vi "Set PCL Decimation.vi"(8 "error in (no error)":errorcluster, 10 "PCL decimation":u32=1, 11 "instrument addon refnum in":T1 format="%.0x") -> (0 "error out":errorcluster, 3 "instrument addon refnum":T1 format="%.0x")   [LabVIEW 2019, in "Instrument Addon Scripting API.lvlib"]
doc: "Assigns a new PCL decimation value to the specified Instrument Addon Custom Device."
uses:
  Instrument Addon Scripting API.lvlib
  <vilib>/NI VeriStand/Custom Device API/Custom Device Item Ref.ctl
  Addon/Addon Shared/SubVIs/Constants.vi
  <vilib>/NI/NI VeriStand Advanced SysDef API/_SubVIs/SysDef.Property.Set.U32.vi
  Addon/Addon Shared/Instrument Addon Shared.lvlib
  <vilib>/NI/NI VeriStand Advanced SysDef API/SysDef API/Advanced System Definition.lvlib
  <vilib>/NI VeriStand/Custom Device API/Custom Device API.lvlib
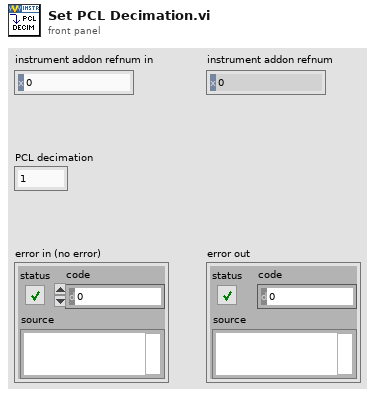
[diagram p1: front panel]
types:
  T1 = typedef "Custom Device API.lvlib/Custom Device Item Ref.ctl" = u64
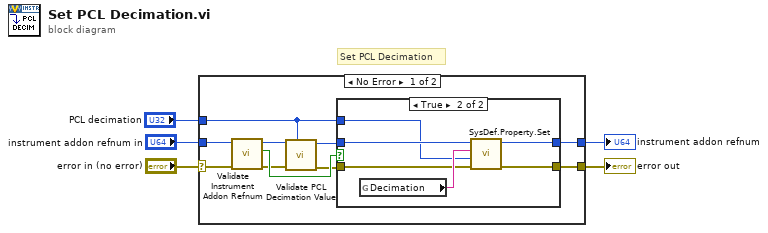
[diagram p0: block diagram]
diagram:
  # "Set PCL Decimation"
  n1 = case shown="No Error" "error in (no error)" {
    selector: "error in (no error)" -> [w11 w25]
    tunnel: "instrument addon refnum in" -> [w10 w24]
    tunnel: [w15 w25] -> w4
    tunnel: [w14 w24] -> w1
    tunnel: "PCL decimation" -> [w12 _]
    frame No Error {
      n2 = call "Validate Instrument Addon Refnum.vi"("Error In"=w11, "Refnum In"=w10) -> ("Error Out"=w8:errorcluster, "Is Instrument Addon?"=w13:bool, "Refnum Out"=w9:T1)  [unwired: 7 in]
      n3 = call "Validate PCL Decimation Value.vi"("PCL Decimation"=w12, "Error In"=w8, "Instrument Addon Refnum In"=w9) -> ("Error Out"=w7:errorcluster, "Instrument Addon Refnum Out"=w6:T1)  [unwired: 7 in]
      n4 = case shown="True" w13 {
        tunnel: w12 -> [_ w18]
        tunnel: [w16 w22] -> w15
        tunnel: [w17 w21] -> w14
        tunnel: w6 -> [w17 w20]
        tunnel: w7 -> [w16 w19]
        frame False {
        }
        frame True {
          n5 = global read "Constants.vi" "Decimation"() -> (w23:string)
          n6 = call-poly <vilib>:"SysDef.Property.Set.vi"("error in (no error)"=w19, "Value"=w18, "Property Name"=w23, "nodeID"=w20) -> ("error out"=w22:errorcluster, "nodeID out"=w21:u64)  [unwired: 6 in]
        }
      }
    }
    frame Error {
    }
  }
  "error out" <- w4
  "instrument addon refnum" <- w1
